vi "R1Master.vi"(6 "LabVIEW Web Service":refnum<class "Web Service.lvclass">) -> ()   [LabVIEW 2016]
uses:
  <vilib>/wsapi/Web Service.lvclass
  R1Controls/R1SBR_SetParams.ctl
  Controls/pH_SetParams Standard.ctl
  <vilib>/Platform/TimedLoop/XDataNode/timing_clust.ctl
  <vilib>/Platform/TimedLoop/XDataNode/nitl_modes.ctl
  <vilib>/Platform/TimedLoop/XDataNode/wakeup.ctl
  <vilib>/Platform/TimedLoop/XDataNode/loadnilvce.vi
  <vilib>/Platform/TimedLoop/XDataNode/XDataNode.xnode
  <vilib>/Platform/TimedLoop/XDataNode/XDNodeRunTimeDep.lvlib
panel:
  out "error out Na":errorcluster
  out "error Out NH4 Nh4":errorcluster
  out "error out":errorcluster
  out "replace with nh4 set params":T1={"Set Point, mg/L"=0.0, "Tolerance, mg/L"=0.05, "N2 Valve Gain"=5000.0, "Air Valve Gain"=1000.0}
  in  "R1NH4Manual":cluster{"NH4 Pump Flowrate, ml/min":dbl}
  out "replace with nh4 switch":bool=TRUE
  in  "R1DOSetParams 2":T1={"Set Point, mg/L"=0.0, "Tolerance, mg/L"=0.05, "N2 Valve Gain"=5000.0, "Air Valve Gain"=1000.0}
  in  "R1 NH4_Switch":bool=TRUE
  out "add NH4 NA probes":cluster{"Signal":dbl, "Value":dbl}
  out "error out (DATA COLLECT)":errorcluster
  out "error out (SBR)":errorcluster
  out "Graph":T2(graph)
  in  "R1SBRManual":T3
  in  "R1SBR_SetParams":T4=[{"Phase"="Plug Feed", "Time, min"=53.0, "SBR_Manual"={"Media Pump"=TRUE, "Water Pump"=TRUE, "Gas Pump"=FALSE, "Effluent Pump"=FALSE}}, {"Phase"="Mixed Feed", "Time, min"=47.0, "SBR_Manual"={"Media Pump"=TRUE, "Water Pump"=TRUE, "Gas Pump"=TRUE, "Effluent Pump"=FALSE}}, {"Phase"="Mixed w/o Feed", "Time, min"=0.0, "SBR_Manual"={"Media Pump"=FALSE, "Water Pump"=FALSE, "Gas Pump"=TRUE, "Effluent Pump"=FALSE}}, {"Phase"="Settle", "Time, min"=5.0, "SBR_Manual"={"Media Pump"=FALSE, "Water Pump"=FALSE, "Gas Pump"=FALSE, "Effluent Pump"=FALSE}}, {"Phase"="Decant", "Time, min"=5.0, "SBR_Manual"={"Media Pump"=FALSE, "Water Pump"=FALSE, "Gas Pump"=FALSE, "Effluent Pump"=TRUE}}, {"Phase"="Idle", "Time, min"=1.0, "SBR_Manual"={"Media Pump"=FALSE, "Water Pump"=FALSE, "Gas Pump"=FALSE, "Effluent Pump"=FALSE}}]
  in  "R1 SBR_Switch":bool=TRUE
  out "R1ORP":T5
  in  "R1DOSetParams":T1={"Set Point, mg/L"=0.0, "Tolerance, mg/L"=0.05, "N2 Valve Gain"=5000.0, "Air Valve Gain"=1000.0}
  in  "R1DOManual":cluster{"Air MFC":dbl, "N2 MFC":dbl} {"Air MFC" scale=0.0..500.0; "N2 MFC" scale=0.0..500.0}
  in  "R1 DO_Switch":bool=TRUE
  out "R1DO":cluster{"Signal":dbl, "Value":dbl}
  in  "R1 pH_Switch":bool=TRUE
  in  "R1pH_SetParams":T6={"Set Point"=7.0, "Tolerance"=0.1, "Pump Time On, secs"=6.0}
  in  "R1pH_Manual":cluster{"Acid Pump":bool, "Base Pump":bool}
  out "pH":cluster{"Signal":dbl, "Value":dbl}
  out "Timestamp":string
  out "Status":string
  out "Cycle Time Elapsed":dbl
  out "Phase Time Elapsed":dbl
  # "Use the web service input terminal to call the VIs on the Service subpalette of the Web Services palette. Do not remove it from the connector pane unless you don't need access to the palette."
  # "Any additional terminals added to the connector pane of a startup VI will be ignored."
  # "SBR Control"
  # "If On, Automate SBR Cycle"
  # "DO Control"
  # "pH Control"
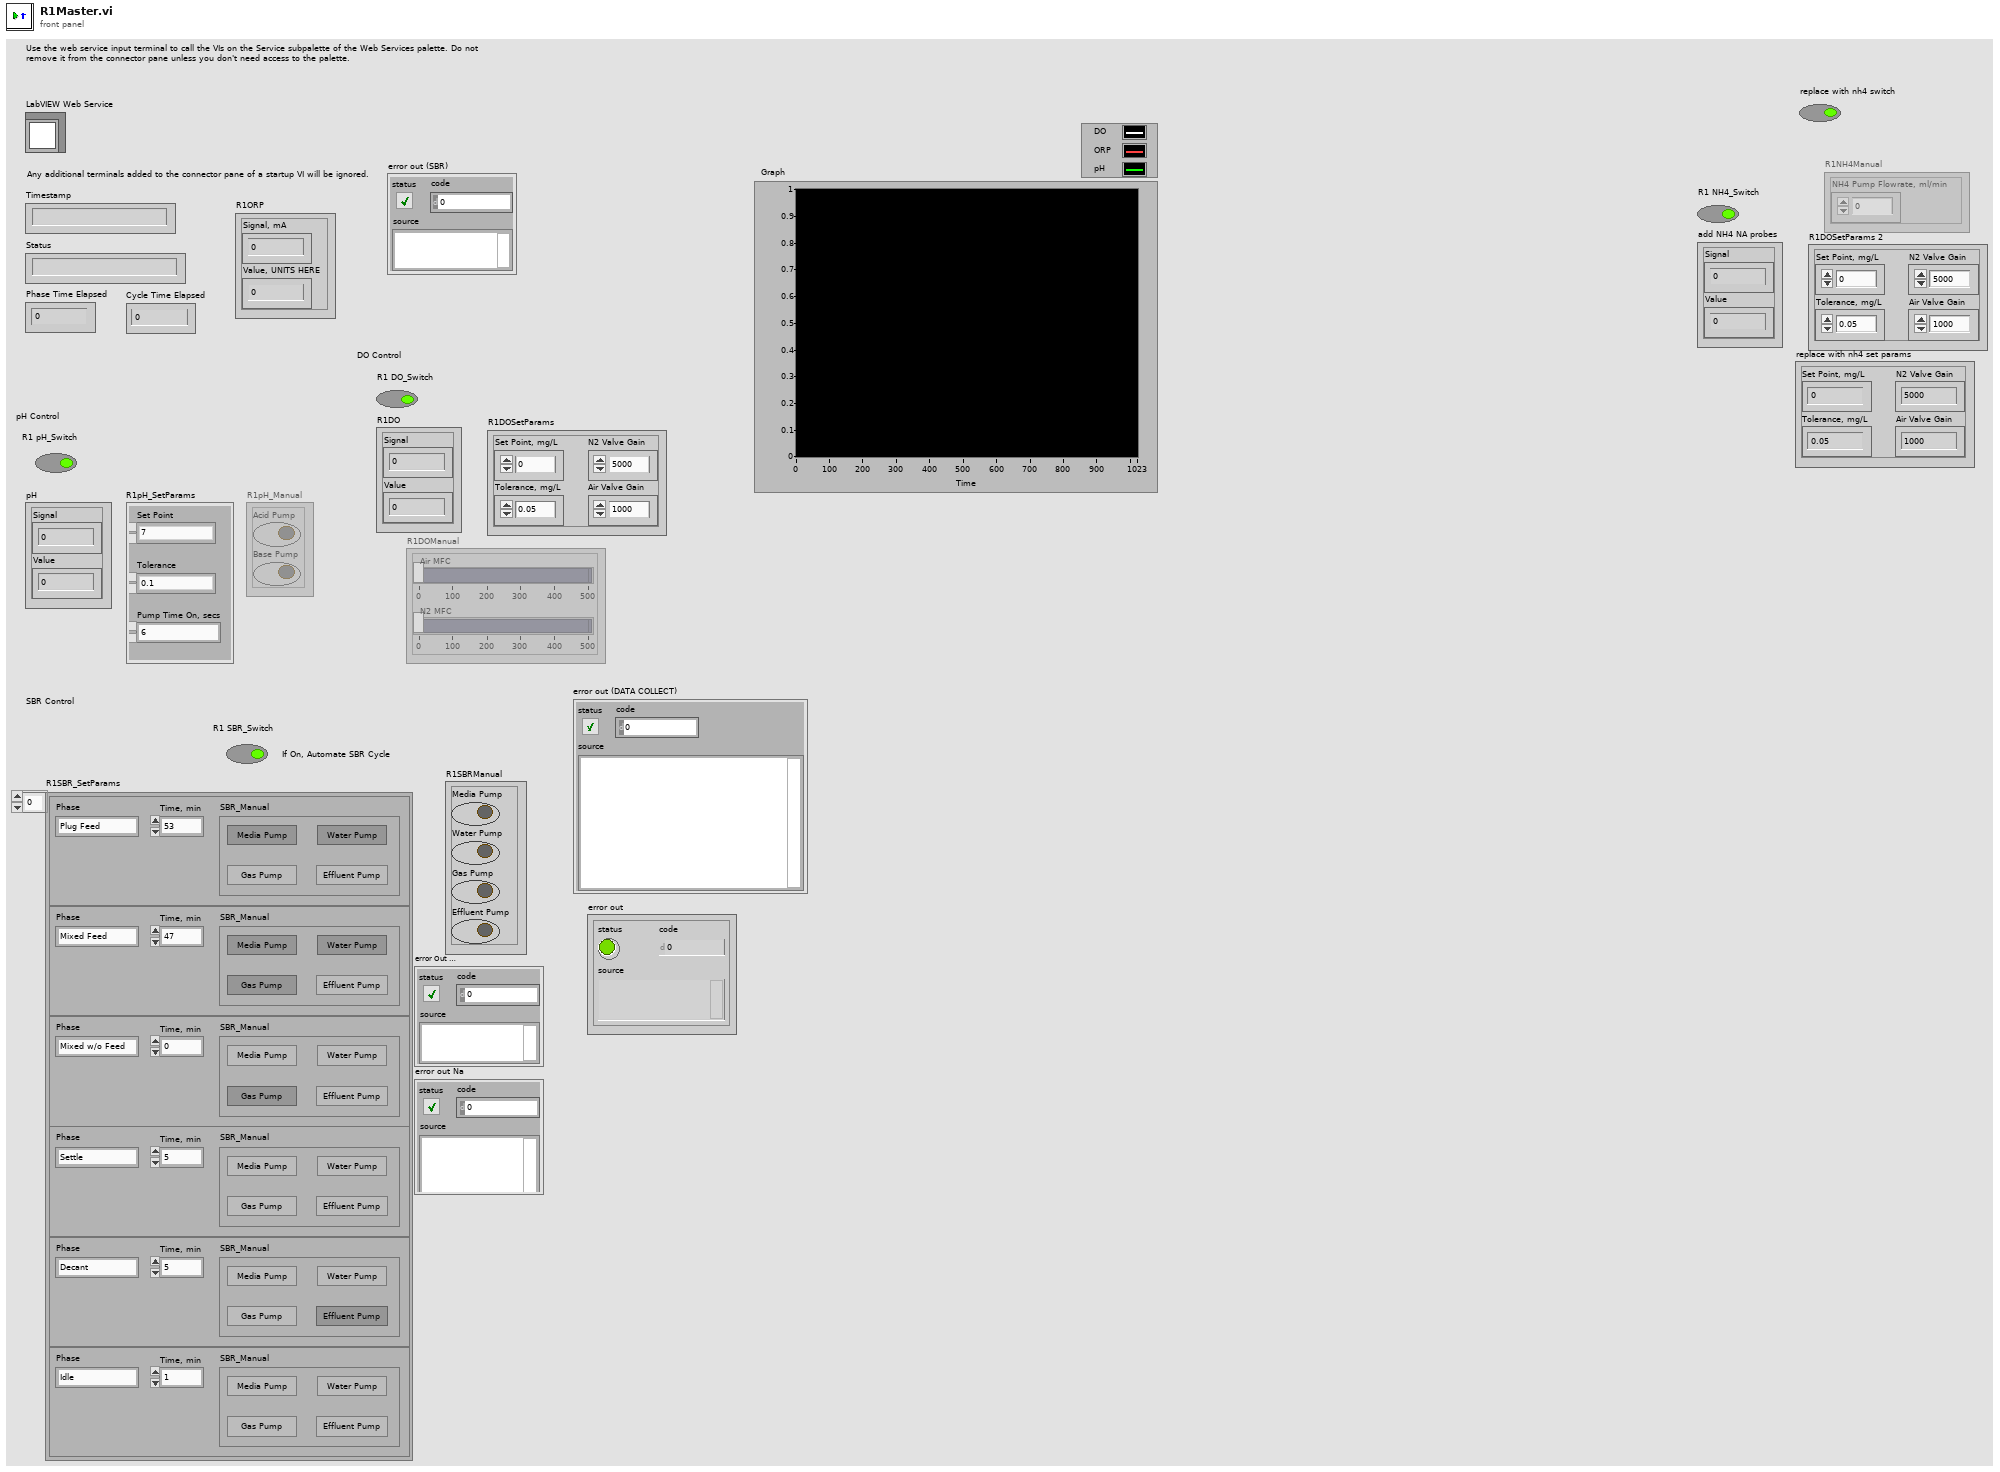
[diagram p1: front panel]
types:
  T1 = cluster{"Set Point, mg/L":dbl, "Tolerance, mg/L":dbl, "N2 Valve Gain":dbl, "Air Valve Gain":dbl}
  T2 = cluster{"Value":dbl, "Value, UNITS HERE":dbl, "Value":dbl}
  T3 = cluster{"Media Pump":bool, "Water Pump":bool, "Gas Pump":bool, "Effluent Pump":bool}
  T4 = typedef "R1SBR_SetParams.ctl" = cluster{"Phase":string, "Time, min":dbl, "SBR_Manual":cluster{"Media Pump":bool, "Water Pump":bool, "Gas Pump":bool, "Effluent Pump":bool}}[]
  T5 = cluster{"Signal, mA":dbl, "Value, UNITS HERE":dbl}
  T6 = typedef "pH_SetParams Standard.ctl" = cluster{"Set Point":dbl, "Tolerance":dbl, "Pump Time On, secs":dbl}
  T7 = typedef "XDNodeRunTimeDep.lvlib/timing_clust.ctl" = cluster{"Expected End [f-1]":u64, "Actual End [f-1]":u64, "Finished Late? [f-1]":bool, "Expected End [i-1]":u64, "Actual End [i-1]":u64, "Finished Late? [i-1]":bool, "Expected Start [i]":u64, "Actual Start [i]":u64, "Expected Start [f]":u64, "Actual Start [f]":u64, "Source Name":string, "Structure Name":string, "Period":i64, "Deadline":i64, "Offset":i64, "Start":i64, "Priority":i32, "Timeout":i32, "Mode":T8, "Wakeup Reason":T9, "Error":errorcluster, "Source Type":string, "Secondary Source Type":string, "Global End Time":u64, "Global Start Time":u64, "Frame Duration":u64, "Iteration Duration":u64, "Assigned CPU":i32, "I/O Scan Engine Mode":u32}
  T8 = typedef "XDNodeRunTimeDep.lvlib/nitl_modes.ctl" = enum32{"No Change", "Process missed periods, maintain original phase", "Discard missed periods, maintain original phase", "Process missed periods, ignore original phase", "Discard missed periods, ignore original phase"}
  T9 = typedef "XDNodeRunTimeDep.lvlib/wakeup.ctl" = enum32{"Normal", "Aborted", "Asynchronous wakeup", "Timing source error", "Timed loop error", "Timeout"}
  T10 = enum8{"Enabled", "Disabled", "Disabled and Grayed Out"}
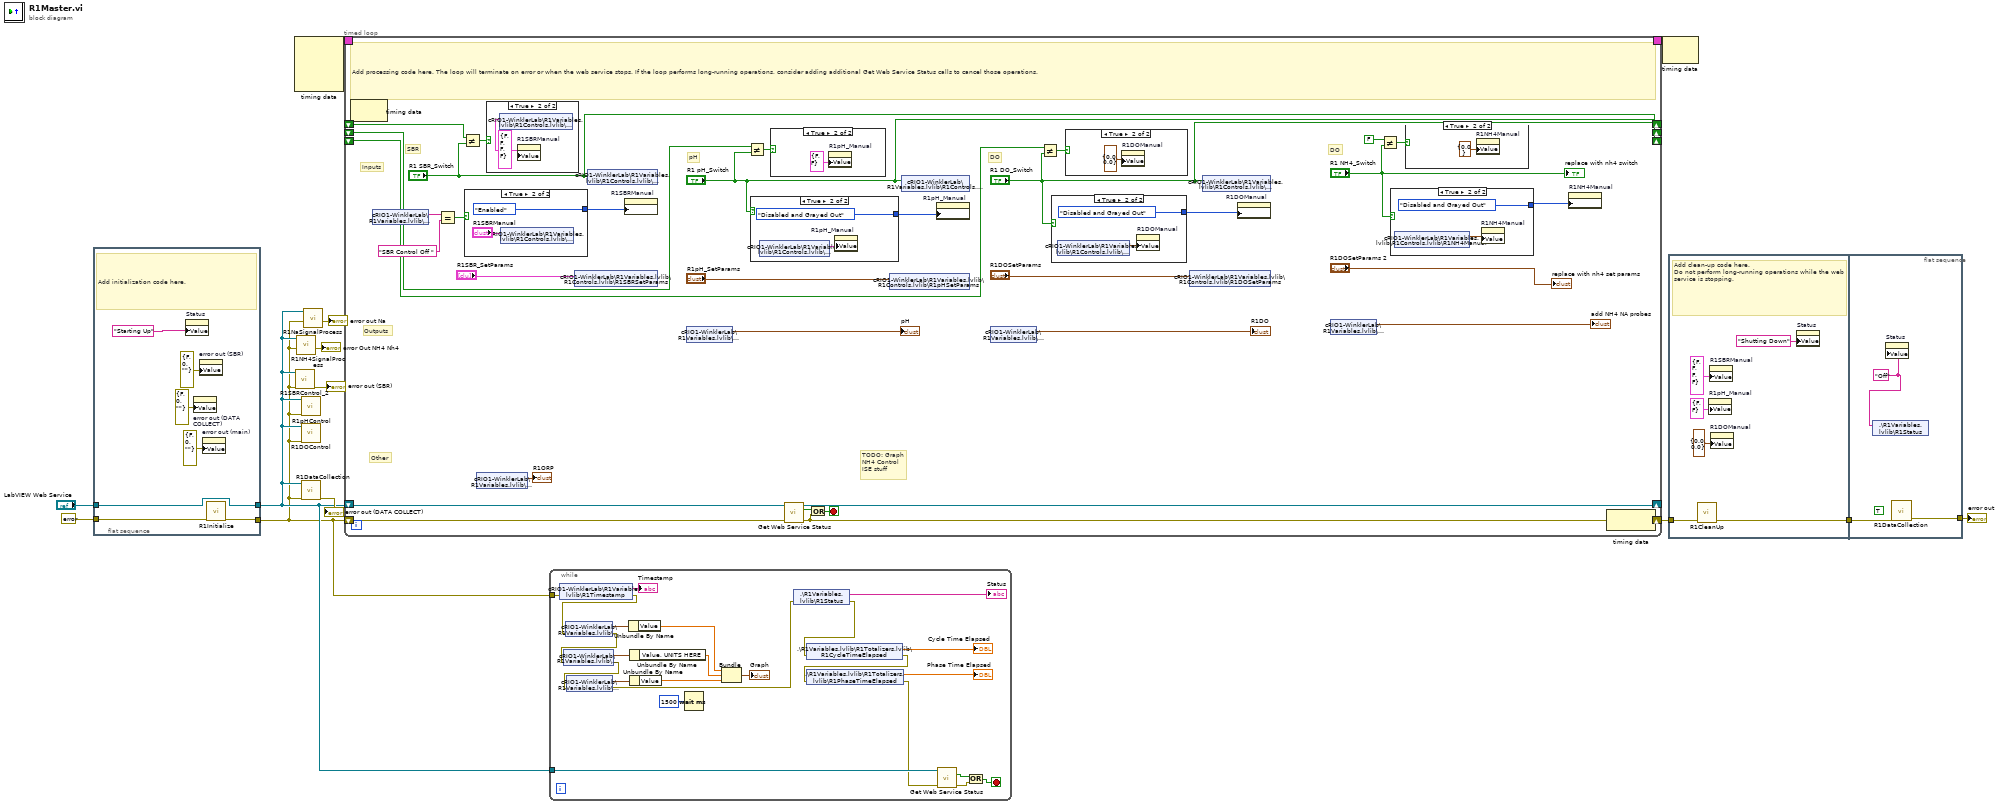
[diagram p0: block diagram]
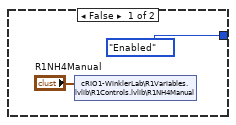
[diagram p3: hidden frame]
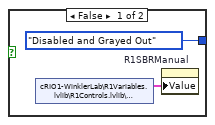
[diagram p7: hidden frame]
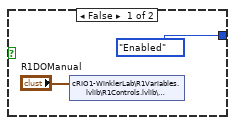
[diagram p8: hidden frame]
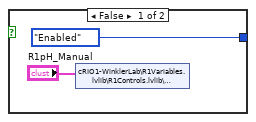
[diagram p9: hidden frame]
diagram:
  n1 = flat-sequence {
    tunnel: "LabVIEW Web Service" -> [w18]
    tunnel: errorcluster {"status"=FALSE, "code"=0, "source"=""} ("error constant") -> [w20]
    tunnel: [w19] -> w3
    tunnel: [w18] -> w4
    frame #0 {
      # "Add initialization code here."
      n2 = property on="Status" class="Str"("Value"="Starting Up" ("Status")) -> ()  [unwired: 2 in, 2 out]
      n3 = property on="error out (DATA COLLECT)" class="Clust (strict)"("Value"=errorcluster {"status"=FALSE, "code"=0, "source"=""} ("error out (DATA COLLECT)")) -> ()  [unwired: 2 in, 2 out]
      n4 = property on="error out (SBR)" class="Clust (strict)"("Value"=errorcluster {"status"=FALSE, "code"=0, "source"=""} ("error out (SBR)")) -> ()  [unwired: 2 in, 2 out]
      n5 = property on="error out (main)" class="Clust (strict)"("Value"=errorcluster {"status"=FALSE, "code"=0, "source"=""} ("error out")) -> ()  [unwired: 2 in, 2 out]
      n6 = call "R1Initialize.vi"("error in (no error)"=w20) -> ("error out"=w19:errorcluster)  [unwired: 10 in]
    }
  }
  n7 = node-c288() -> (w10:T7)  [unwired: 4 in]
  n8 = call "R1SBRControl_2.vi"("error constant"=w3, "LabVIEW Web Service"=w4) -> ("error out"=→"error out (SBR)":errorcluster)  [unwired: 9 in]
  n9 = call "R1NH4SignalProcess.vi"("error"=w3, "LabVIEW Web Service"=w4) -> ("error Out"=→"error Out NH4 Nh4":errorcluster)  [unwired: 9 in]
  n10 = call "R1pHControl.vi"("error constant"=w3, "LabVIEW Web Service"=w4) -> ()  [unwired: 10 in]
  n11 = call "R1DOControl.vi"("error constant"=w3, "LabVIEW Web Service"=w4) -> ()  [unwired: 10 in]
  n12 = call "R1DataCollection.vi"("error constant"=w3, "LabVIEW Web Service"=w4) -> ("error out"=→"error out (DATA COLLECT)":errorcluster)  [unwired: 9 in]
  n13 = call "R1NaSignalProcess.vi"("error"=w3, "LabVIEW Web Service"=w4) -> ("error out"=→"error out Na":errorcluster)  [unwired: 9 in]
  n14 = timed-loop {
    shift-right: [w51] -> w11
    shift-left: w3 -> [w50]
    shift-right: [w47] -> _
    shift-left: w4 -> [w47]
    timing: w10 -> [_]
    timing-out: [_] -> w9
    shift-right: ["R1 SBR_Switch"] -> _
    shift-left: _ -> [w21]
    shift-right: ["R1 pH_Switch"] -> _
    shift-left: _ -> [w36]
    shift-right: ["R1 DO_Switch"] -> _
    shift-left: _ -> [w34]
    stop <- w49 stop-if-true
    # "DO"
    # "TODO: Graph\nNH4 Control\nISE stuff"
    # "DO"
    # "pH"
    # "Other"
    # "Outputs"
    # "Inputs"
    # "SBR"
    # "Add processing code here. The loop will terminate on error or when the web service stops. If the loop performs long-running operations, consider adding additional Get Web Service Status calls to cancel those operations."
    n15 = node-c288() -> ()  [unwired: 1 in, 1 out]
    n16 = shared-variable "cRIO1-WinklerLab\\R1Variables.lvlib\\R1Status"() -> (w24:string)  [unwired: 1 in, 1 out]
    n17 = Equal?(x=w24, y="SBR Control Off " ("string")) -> (x = y?=w22:bool)
    n18 = Not Equal?(x=w21, y="R1 SBR_Switch") -> (x != y?=w38:bool)
    n19 = case shown="True" w22 {
      tunnel: [T10."Disabled and Grayed Out" ("Disabled") T10."Enabled" ("Disabled")] -> w39
      frame False {
        n20 = shared-variable "cRIO1-WinklerLab\\R1Variables.lvlib\\R1Controls.lvlib\\R1SBRManual"() -> (w61:T3)  [unwired: 1 in, 1 out]
        n21 = property on="R1SBRManual" class="Clust (strict)"("Value"=w61) -> ()  [unwired: 2 in, 2 out]
      }
      frame True {
        n22 = shared-variable "cRIO1-WinklerLab\\R1Variables.lvlib\\R1Controls.lvlib\\R1SBRManual"("R1SBRManual") -> ()  [unwired: 1 in, 1 out]
      }
    }
    n23 = shared-variable "cRIO1-WinklerLab\\R1Variables.lvlib\\R1Signals.lvlib\\R1ORP"() -> (→"R1ORP":T5)  [unwired: 1 in, 1 out]
    n24 = case shown="True" w38 {
      frame False {
      }
      frame True {
        w60 = T3 {"Media Pump"=FALSE, "Water Pump"=FALSE, "Gas Pump"=FALSE, "Effluent Pump"=FALSE} ("R1SBRManual")
        n25 = shared-variable "cRIO1-WinklerLab\\R1Variables.lvlib\\R1Controls.lvlib\\R1SBRManual"(w60) -> ()  [unwired: 1 in, 1 out]
        n26 = property on="R1SBRManual" class="Clust (strict)"("Value"=w60) -> ()  [unwired: 2 in, 2 out]
      }
    }
    n27 = shared-variable "cRIO1-WinklerLab\\R1Variables.lvlib\\R1Controls.lvlib\\R1SBRSetParams"("R1SBR_SetParams") -> ()  [unwired: 1 in, 1 out]
    n28 = shared-variable "cRIO1-WinklerLab\\R1Variables.lvlib\\R1Controls.lvlib\\R1SBRSwitch"("R1 SBR_Switch") -> ()  [unwired: 1 in, 1 out]
    n29 = property on="R1SBRManual" class="Clust (strict)"("DisabledEnum"=w39) -> ()  [unwired: 2 in, 2 out]
    n30 = shared-variable "cRIO1-WinklerLab\\R1Variables.lvlib\\R1Signals.lvlib\\R1pH"() -> (→"pH":cluster{"Signal":dbl, "Value":dbl})  [unwired: 1 in, 1 out]
    n31 = Not Equal?(x=w36, y="R1 pH_Switch") -> (x != y?=w35:bool)
    n32 = case shown="True" "R1 pH_Switch" {
      tunnel: [T10."Enabled" ("Disabled") T10."Disabled and Grayed Out" ("Disabled")] -> w45
      frame False {
        n33 = shared-variable "cRIO1-WinklerLab\\R1Variables.lvlib\\R1Controls.lvlib\\R1pHManual"("R1pH_Manual") -> ()  [unwired: 1 in, 1 out]
      }
      frame True {
        n34 = shared-variable "cRIO1-WinklerLab\\R1Variables.lvlib\\R1Controls.lvlib\\R1pHManual"() -> (w71:cluster{"Acid Pump":bool, "Base Pump":bool})  [unwired: 1 in, 1 out]
        n35 = property on="R1pH_Manual" class="Clust (strict)"("Value"=w71) -> ()  [unwired: 2 in, 2 out]
      }
    }
    n36 = case shown="True" w35 {
      frame False {
      }
      frame True {
        n37 = property on="R1pH_Manual" class="Clust (strict)"("Value"=cluster{"Acid Pump":bool, "Base Pump":bool} {"Acid Pump"=FALSE, "Base Pump"=FALSE} ("R1pH_Manual")) -> ()  [unwired: 2 in, 2 out]
      }
    }
    n38 = call <vilib>:"Get Web Service Status.vi"("LabVIEW Web Service"=w47, "error in (no error)"=w50) -> ("service stopping?"=w52:bool, "error out"=w51:errorcluster)  [unwired: 11 in, 1 out]
    n39 = Or(x=w52, y=w51) -> (x .or. y?=w49:bool)
    n40 = shared-variable "cRIO1-WinklerLab\\R1Variables.lvlib\\R1Controls.lvlib\\R1pHSetParams"("R1pH_SetParams") -> ()  [unwired: 1 in, 1 out]
    n41 = shared-variable "cRIO1-WinklerLab\\R1Variables.lvlib\\R1Controls.lvlib\\R1pHSwitch"("R1 pH_Switch") -> ()  [unwired: 1 in, 1 out]
    n42 = property on="R1pH_Manual" class="Clust (strict)"("DisabledEnum"=w45) -> ()  [unwired: 2 in, 2 out]
    n43 = shared-variable "cRIO1-WinklerLab\\R1Variables.lvlib\\R1Signals.lvlib\\R1DO"() -> (→"R1DO":cluster{"Signal":dbl, "Value":dbl})  [unwired: 1 in, 1 out]
    n44 = Not Equal?(x=w34, y="R1 DO_Switch") -> (x != y?=w33:bool)
    n45 = case shown="True" "R1 DO_Switch" {
      tunnel: [T10."Enabled" ("Disabled") T10."Disabled and Grayed Out" ("Disabled")] -> w42
      frame False {
        n46 = shared-variable "cRIO1-WinklerLab\\R1Variables.lvlib\\R1Controls.lvlib\\R1DOManual"("R1DOManual") -> ()  [unwired: 1 in, 1 out]
      }
      frame True {
        n47 = shared-variable "cRIO1-WinklerLab\\R1Variables.lvlib\\R1Controls.lvlib\\R1DOManual"() -> (w67:cluster{"Air MFC":dbl, "N2 MFC":dbl})  [unwired: 1 in, 1 out]
        n48 = property on="R1DOManual" class="Clust (strict)"("Value"=w67) -> ()  [unwired: 2 in, 2 out]
      }
    }
    n49 = case shown="True" w33 {
      frame False {
      }
      frame True {
        n50 = property on="R1DOManual" class="Clust (strict)"("Value"=cluster{"Air MFC":dbl, "N2 MFC":dbl} {"Air MFC"=0.0, "N2 MFC"=0.0} ("R1DOManual")) -> ()  [unwired: 2 in, 2 out]
      }
    }
    n51 = shared-variable "cRIO1-WinklerLab\\R1Variables.lvlib\\R1Controls.lvlib\\R1DOSetParams"("R1DOSetParams") -> ()  [unwired: 1 in, 1 out]
    n52 = shared-variable "cRIO1-WinklerLab\\R1Variables.lvlib\\R1Controls.lvlib\\R1DOSwitch"("R1 DO_Switch") -> ()  [unwired: 1 in, 1 out]
    n53 = property on="R1DOManual" class="Clust (strict)"("DisabledEnum"=w42) -> ()  [unwired: 2 in, 2 out]
    n54 = shared-variable "cRIO1-WinklerLab\\R1Variables.lvlib\\R1Signals.lvlib\\R1DO"() -> (→"add NH4 NA probes":cluster{"Signal":dbl, "Value":dbl})  [unwired: 1 in, 1 out]
    n55 = Not Equal?(x=FALSE, y="R1 NH4_Switch") -> (x != y?=w30:bool)
    n56 = case shown="True" "R1 NH4_Switch" {
      tunnel: [T10."Enabled" ("Disabled") T10."Disabled and Grayed Out" ("Disabled")] -> w26
      frame False {
        n57 = shared-variable "cRIO1-WinklerLab\\R1Variables.lvlib\\R1Controls.lvlib\\R1NH4Manual"("R1NH4Manual") -> ()  [unwired: 1 in, 1 out]
      }
      frame True {
        n58 = shared-variable "cRIO1-WinklerLab\\R1Variables.lvlib\\R1Controls.lvlib\\R1NH4Manual"() -> (w56:cluster{"NH4 Pump Flowrate, ml/min":dbl})  [unwired: 1 in, 1 out]
        n59 = property on="R1NH4Manual" class="Clust (strict)"("Value"=w56) -> ()  [unwired: 2 in, 2 out]
      }
    }
    n60 = case shown="True" w30 {
      frame False {
      }
      frame True {
        n61 = property on="R1NH4Manual" class="Clust (strict)"("Value"=cluster{"NH4 Pump Flowrate, ml/min":dbl} {"NH4 Pump Flowrate, ml/min"=0.0} ("R1NH4Manual")) -> ()  [unwired: 2 in, 2 out]
      }
    }
    n62 = property on="R1NH4Manual" class="Clust (strict)"("DisabledEnum"=w26) -> ()  [unwired: 2 in, 2 out]
    n63 = node-c288() -> ()  [unwired: 1 in, 1 out]
    "replace with nh4 switch" <- "R1 NH4_Switch"
    "replace with nh4 set params" <- "R1DOSetParams 2"
  }
  n64 = while {
    tunnel: w4 -> [w91]
    tunnel: w3 -> [w82]
    stop <- w88 stop-if-true
    n65 = shared-variable "cRIO1-WinklerLab\\R1Variables.lvlib\\R1Timestamp"(error in=w82) -> (→"Timestamp":string, error out=w81:errorcluster)
    n66 = shared-variable "cRIO1-WinklerLab\\R1Variables.lvlib\\R1Signals.lvlib\\R1DO"(error in=w81) -> (w92:cluster{"Signal":dbl, "Value":dbl}, error out=w80:errorcluster)
    n67 = shared-variable "cRIO1-WinklerLab\\R1Variables.lvlib\\R1Signals.lvlib\\R1ORP"(error in=w80) -> (w93:T5, error out=w79:errorcluster)
    n68 = shared-variable "cRIO1-WinklerLab\\R1Variables.lvlib\\R1Signals.lvlib\\R1pH"(error in=w79) -> (w94:cluster{"Signal":dbl, "Value":dbl}, error out=w78:errorcluster)
    n69 = Unbundle By Name(w92) -> ("Value"=w95:dbl)
    n70 = Unbundle By Name(w93) -> ("Value, UNITS HERE"=w96:dbl)
    n71 = Unbundle By Name(w94) -> ("Value"=w97:dbl)
    n72 = Wait (ms)(milliseconds to wait=u32 1500) -> ()  [unwired: 1 out]
    n73 = Bundle("Value"=w95, "Value, UNITS HERE"=w96, "Value"=w97) -> (→"Graph":T2)  [unwired: 1 in]
    n74 = shared-variable ".\\R1Variables.lvlib\\R1Status"(error in=w78) -> (→"Status":string, error out=w77:errorcluster)
    n75 = shared-variable ".\\R1Variables.lvlib\\R1Totalizers.lvlib\\R1CycleTimeElapsed"(error in=w77) -> (→"Cycle Time Elapsed":dbl, error out=w76:errorcluster)
    n76 = shared-variable ".\\R1Variables.lvlib\\R1Totalizers.lvlib\\R1PhaseTimeElapsed"(error in=w76) -> (→"Phase Time Elapsed":dbl, error out=w75:errorcluster)
    n77 = call <vilib>:"Get Web Service Status.vi"("LabVIEW Web Service"=w91, "error in (no error)"=w75) -> ("service stopping?"=w90:bool, "error out"=w89:errorcluster)  [unwired: 11 in, 1 out]
    n78 = Or(x=w90, y=w89) -> (x .or. y?=w88:bool)
  }
  n79 = node-c288(w9) -> ()  [unwired: 1 out]
  n80 = flat-sequence {
    tunnel: w11 -> [w101]
    tunnel: [w100] -> w7
    tunnel: w7 -> [w107]
    tunnel: [w106] -> w6
    frame #0 {
      # "Add clean-up code here.\nDo not perform long-running operations while the web service is stopping."
      n81 = call "R1CleanUp.vi"("error in (no error)"=w101) -> ("error out"=w100:errorcluster)  [unwired: 10 in]
      n82 = property on="R1pH_Manual" class="Clust (strict)"("Value"=cluster{"Acid Pump":bool, "Base Pump":bool} {"Acid Pump"=FALSE, "Base Pump"=FALSE} ("R1pH_Manual")) -> ()  [unwired: 2 in, 2 out]
      n83 = property on="R1SBRManual" class="Clust (strict)"("Value"=T3 {"Media Pump"=FALSE, "Water Pump"=FALSE, "Gas Pump"=FALSE, "Effluent Pump"=FALSE} ("R1SBRManual")) -> ()  [unwired: 2 in, 2 out]
      n84 = property on="R1DOManual" class="Clust (strict)"("Value"=cluster{"Air MFC":dbl, "N2 MFC":dbl} {"Air MFC"=0.0, "N2 MFC"=0.0} ("R1DOManual")) -> ()  [unwired: 2 in, 2 out]
      n85 = property on="Status" class="Str"("Value"="Shutting Down" ("Status")) -> ()  [unwired: 2 in, 2 out]
    }
    frame #1 {
      w105 = "Off" ("Status")
      (unwired) TRUE ("Write Once")
      n86 = shared-variable ".\\R1Variables.lvlib\\R1Status"(w105) -> ()  [unwired: 1 in, 1 out]
      n87 = property on="Status" class="Str"("Value"=w105) -> ()  [unwired: 2 in, 2 out]
      n88 = call "R1DataCollection.vi"("error constant"=w107) -> ("error out"=w106:errorcluster)  [unwired: 10 in]
    }
  }
  "error out" <- w6
